vi "DS345_BurstMode.constructor.vi"(0 "name":string, 2 "data in":string, 5 "error in (no error)":errorcluster) -> (14 "i ref out":refnum<vi>, 16 "data out":string, 19 "error out":errorcluster)   [LabVIEW 2014, in "DS345_BurstMode.lvlib"]
doc: "Constructor of the DS345 class.\n\nauthor: Dietrich Beck, GSI\nmaintainer: Dietrich Beck, GSI\n\nLicense Agreement for this software:\n\nCopyright (C)\nGesellschaft für Schwerionenforschung, GSI\nPlanckstr. 1\n64291 Darmstadt\nGermany\n\nContact: D.Beck@gsi.de \n\nThis program is free software; you can redistribute it and/or modify it under the terms of the \nGNU General Public License as published by the Free Software Foundation; either version 2 of \nthe license, or (at your option) any later version.\n\nThis program is distributed in the hope that it will be useful, but WITHOUT ANY WARRANTY; \nwithout even the implied warranty of MERCHANTABILITY or FITNESS FOR A PARTICULAR PURPOSE. See the GNU General License for more details (http://www.gnu.org).\n\nGesellschaft für Schwerionenforschung, GSI\nPlanckstr. 1, 64291 Darmstadt, Germany\nFor all questions and ideas contact: M.Richter@gsi.de, H.Brand@gsi.de or D.Beck@gsi.de.\nLast update: 16-JUN-2004"
uses:
  DS345_BurstMode.lvlib
  CSCore/CSSystem/CSSystemLib/CSSystemLib.lvlib
  CSCore/CSApplicationBaseClasses/AFGBase/AFGBase.lvlib
  CSCore/CSApplicationBaseClasses/DeviceBase/DeviceBase.lvlib
  CSCore/CSApplicationBaseClasses/DeviceBase/DeviceBase.myEventNames.ctl
  CSCore/CSApplicationBaseClasses/AFGBase/AFGBase.myEventNames.ctl
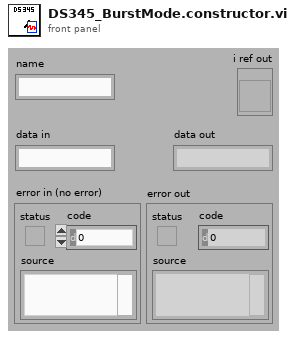
[diagram p1: front panel]
types:
  T1 = enum16{"SetAttribute", "GetAttribute", "CreateAttribute", "DestroyAttribute", "DestroyAllAtributes"}
  T2 = typedef "AFGBase.lvlib/AFGBase.myEventNames.ctl" = enum16{"lvmsg://SetFrequency", "lvmsg://GetFrequency", "lvmsg://SetAmplitude", "lvmsg://GetAmplitude", "lvmsg://SetPhase", "lvmsg://GetPhase", "lvmsg://SetDCOffset", "lvmsg://GetDCOffset", "lvmsg://SetWaveformType", "lvmsg://GetWaveformType", "lvmsg://SetOutputEnabled", "lvmsg://GetOutputEnabled", "lvmsg://SetWaveform", "lvmsg://GetWaveform", "lvmsg://SetTrigger", "lvmsg://GetTrigger", "lvmsg://SetWaveformParams", "lvmsg://GetWaveformParams"}
  T3 = typedef "DeviceBase.lvlib/DeviceBase.myEventNames.ctl" = enum16{"lvmsg://Initialize", "lvmsg://Close", "lvmsg://Configure", "lvmsg://Reset", "lvmsg://IDQuery"}
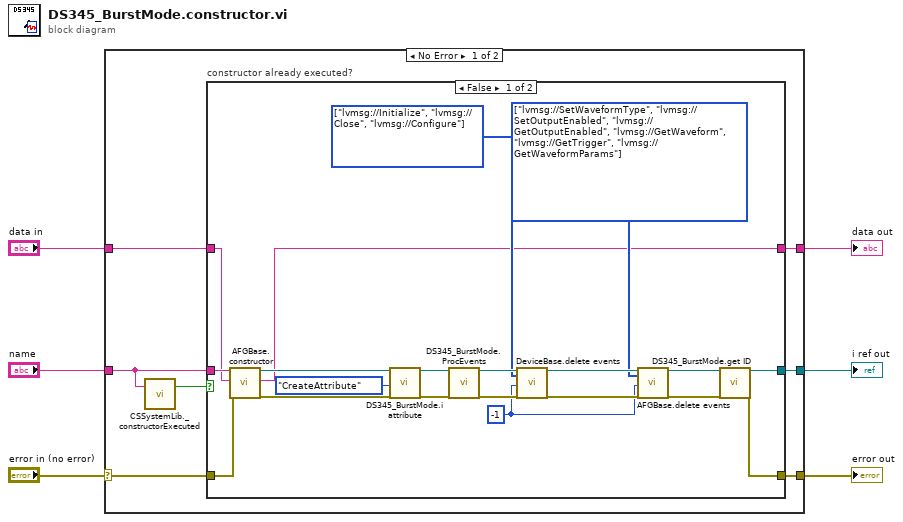
[diagram p0: block diagram]
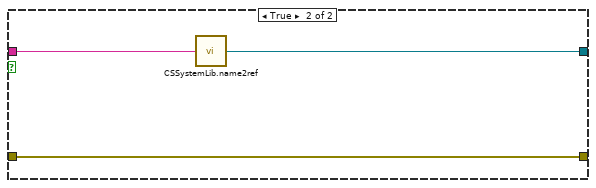
[diagram p2: hidden frame]
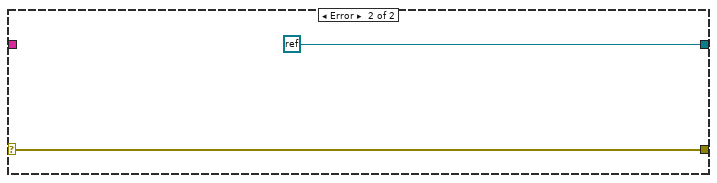
[diagram p3: hidden frame]
diagram:
  n1 = case shown="No Error" "error in (no error)" {
    selector: "error in (no error)" -> [w11 w37]
    tunnel: "name" -> [w10 _]
    tunnel: [w13 refnum<k0> refnum] -> w5
    tunnel: [w12 w37] -> w4
    tunnel: "data in" -> [w8 _]
    tunnel: [w7 _] -> w1
    frame No Error {
      n2 = call "CSSystemLib._constructorExecuted.vi"("name"=w10) -> ("constructor executed?"=w9:bool)  [unwired: 18 in]
      n3 = case "constructor already executed?" shown="False" w9 {
        tunnel: w10 -> [w30 w36]
        tunnel: [w17 w35] -> w13
        tunnel: [w15 w34] -> w12
        tunnel: w11 -> [w27 w34]
        tunnel: w8 -> [w26 _]
        tunnel: [w14 _] -> w7
        frame False {
          w19 = T2[] [enum."lvmsg://SetWaveformType", enum."lvmsg://SetOutputEnabled", enum."lvmsg://GetOutputEnabled", enum."lvmsg://GetWaveform", enum."lvmsg://GetTrigger", enum."lvmsg://GetWaveformParams"] items=["lvmsg://SetFrequency", "lvmsg://GetFrequency", "lvmsg://SetAmplitude", "lvmsg://GetAmplitude", "lvmsg://SetPhase", "lvmsg://GetPhase", "lvmsg://SetDCOffset", "lvmsg://GetDCOffset", "lvmsg://SetWaveformType", "lvmsg://GetWaveformType", "lvmsg://SetOutputEnabled", "lvmsg://GetOutputEnabled", "lvmsg://SetWaveform", "lvmsg://GetWaveform", "lvmsg://SetTrigger", "lvmsg://GetTrigger", "lvmsg://SetWaveformParams", "lvmsg://GetWaveformParams"] ("events")
          w23 = T3[] [enum."lvmsg://Initialize", enum."lvmsg://Close", enum."lvmsg://Configure"] items=["lvmsg://Initialize", "lvmsg://Close", "lvmsg://Configure", "lvmsg://Reset", "lvmsg://IDQuery"] ("events")
          w20 = -1 ("ms timeout (10000)")
          n4 = call "AFGBase.constructor.vi"("name"=w30, "data in"=w26, "error in (no error)"=w27) -> ("i ref out"=w33:refnum<vi>, "data out"=w14:string, "error out"=w32:errorcluster)  [unwired: 14 in]
          n5 = call "DS345_BurstMode.i attribute.vi"("VI Refnum"=w33, "Action"=T1."CreateAttribute", "error in (no error)"=w32) -> ("VI Refnum out"=w29:refnum<vi>, "error out"=w28:errorcluster)  [unwired: 14 in, 1 out]
          n6 = call "DS345_BurstMode.ProcEvents.vi"("i ref in"=w29, "error in (no error)"=w28) -> ("i ref out"=w25:refnum<vi>, "error out"=w24:errorcluster)  [unwired: 16 in]
          n7 = call "DeviceBase.delete events.vi"("i ref in"=w25, "events"=w23, "ms timeout (10000)"=w20, "error in (no error)"=w24) -> ("i ref out"=w22:refnum<vi>, "error out"=w21:errorcluster)  [unwired: 13 in, 1 out]
          n8 = call "AFGBase.delete events.vi"("i ref in"=w22, "events"=w19, "ms timeout (10000)"=w20, "error in (no error)"=w21) -> ("i ref out"=w18:refnum<vi>, "error out"=w16:errorcluster)  [unwired: 13 in, 1 out]
          n9 = call "DS345_BurstMode.get ID.vi"("i ref in"=w18, "error in (no error)"=w16) -> ("i ref out"=w17:refnum<vi>, "error out"=w15:errorcluster)  [unwired: 15 in, 1 out]
        }
        frame True {
          n10 = call "CSSystemLib.name2ref.vi"("name"=w36) -> ("obj refnum"=w35:refnum<vi>)
        }
      }
    }
    frame Error {
    }
  }
  "i ref out" <- w5
  "error out" <- w4
  "data out" <- w1
